vi "Save.vi"(8 "error in (no error)":errorcluster, 11 "PrefsDB in (Singleton)":refnum<class "PrefsDB.lvclass">) -> (0 "error out":errorcluster, 3 "PrefsDB out":refnum<class "PrefsDB.lvclass">)   [LabVIEW 2020, in "User Prefs.lvlib" / "PrefsDB.lvclass"]
uses:
  PrefsDB.lvclass
  Is Valid.vi
  Obtain UserPrefs.vi
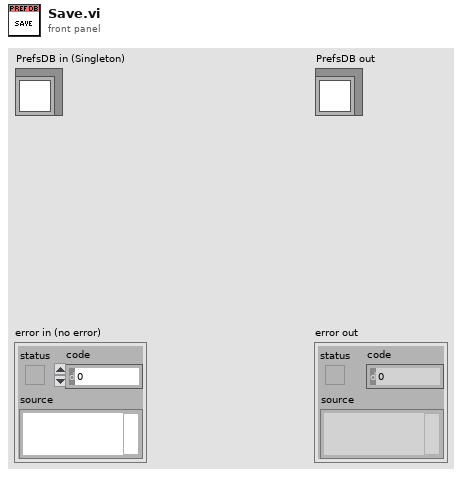
[diagram p1: front panel]
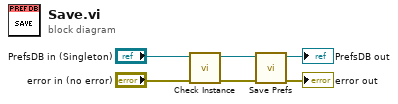
[diagram p0: block diagram]
diagram:
  n1 = call "Check Instance.vi"("error in (no error)"="error in (no error)", "PrefsDB in"="PrefsDB in (Singleton)") -> ("error out"=w2:errorcluster, "PrefsDB out"=w1:refnum<class "PrefsDB.lvclass">)  [unwired: 8 in]
  n2 = call "Save Prefs.vi"("error in (no error)"=w2, "PrefsDB in"=w1) -> ("error out"=→"error out":errorcluster, "PrefsDB out"=→"PrefsDB out":refnum<class "PrefsDB.lvclass">)  [unwired: 8 in]
